vi "Create.vi"   [LabVIEW 2020, in "feature_detection.lvlib" / "WeChat QR Code Detector.lvclass"]
uses:
  WeChat QR Code Detector.lvclass
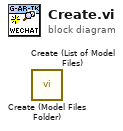
[diagram p0: block diagram]
diagram:
  n1 = call "Create (Model Files Folder).vi"() -> ()  [unwired: 10 in, 2 out]
  n2 = call "Create (List of Model Files).vi"() -> ()  [unwired: 10 in, 2 out]
